vi "Set temperature.vi"(8 "error in (no error)":errorcluster, 10 "temperature (°C)":i16, 11 "camera handle in":i16) -> (0 "error out":errorcluster, 3 "camera handle out":i16)   [LabVIEW 2012]
uses:
  Visual Studio/Cascade wrapper/Release/Cascade wrapper.dll
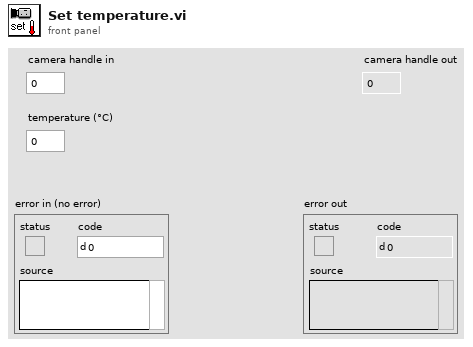
[diagram p1: front panel]
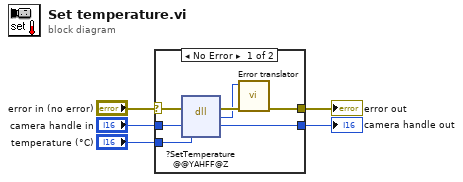
[diagram p0: block diagram]
diagram:
  n1 = case shown="No Error" "error in (no error)" {
    selector: "error in (no error)" -> [w12 w14]
    tunnel: "camera handle in" -> [w11 w13]
    tunnel: "temperature (°C)" -> [w10 _]
    tunnel: [w7 w13] -> w2
    tunnel: [w6 w14] -> w1
    frame No Error {
      n2 = dll-call lib="C:/moroder/Cascade wrapper/Visual Studio/Cascade wrapper/Release/Cascade wrapper.dll" fn="?SetTemperature@@YAHFF@Z"(error in=w12, "camera handle"=w11, "temperature"=w10) -> (error out=w9:errorcluster, "error"=w8:i32, "camera handle"=w7:i16)  [unwired: 3 in, 1 out]
      n3 = call "Error translator.vi"("error in (no error)"=w9, "error code"=w8) -> ("error out"=w6:errorcluster)  [unwired: 9 in]
    }
    frame Error {
    }
  }
  "error out" <- w1
  "camera handle out" <- w2
